vi "CheckTotalSamples.vi"(0 "Digitizer Settings":T1={"Digitizer delay (us) "=0.0, "rf points per line"=0, "lines per plane"=0, "Samp Rate (Hz)"=0.0, "Additional dig delay (us)"=0.0, "Voltage Scale"=0.0, "Pre-Looks"=0, "Offset delay (us)"=0.0, "bits A/D"=0, "Avg Num"=0, "DigTimeOut"=0.0, "Rel Dig Delay"=0.0, "Dig Ch"=0, "LeCroyCluster"={"LeCroy Channels"=[], "LC read pt offset"=0.0, "Sweep Avg"=FALSE}, "Main Digitizer"=enum."Acqiris Digitizer", "Dig Config"=enum."Single channel", "Digitizer ID Cluster"={"Acqiris/Alazar/SP ID"=[], "NI Instr Handles"=[], "LeCroy VISA"="", "GaGe Handle"={"Handle"=0, "Sample size"=0, "Resolution"=0, "Offset"=0, "Channels"=0, "Boards"=0}, "ATS Ref"="ATS9350", "Acqiris Address"=["PCI::INSTR0"], "ADQRef"=refnum, "adq_cu_ptr"=refnum}, "Trigger Settings"={"Trig Source"=1, "Trig Coupling"=0, "Trig Slope"=0, "Level (mV)"=1500.0}, "Bulk Acq"=FALSE, "Bulk Start Indexes"=[], "Data Ref RF"=refnum, "NI ID/Channel"=[], "Total Dig CH"=1, "Xtra Ann Trig delay (us)"=10.0, "Fix Z Delay?"=FALSE, "One Way Transmission?"=FALSE, "Data Ref Log"=refnum} {"Trigger Settings"."Trig Slope" items=["Positive", "Negative"]; "Trigger Settings"."Level (mV)" format="%.2f"; "Trigger Settings"."Trig Coupling" items=["DC 1 MOhm", "AC 1 MOhm", "DC 50 Ohm", "AC 50 Ohm"]; "Trigger Settings"."Trig Source" items=["Chan 1", "External"]; "Rel Dig Delay" format="%.2f"; "DigTimeOut" format="%.2f"; "Avg Num" min=1; "Offset delay (us)" format="%.2f"; "Additional dig delay (us)" format="%.2f"; "Digitizer delay (us)" format="%.2f"}, 1 "Multi Trig":bool, 2 "Multi Trig#":i32, 7 "Valid combo":bool=TRUE, 11 "Bulk Acq":bool) -> (4 "Total Pts":bool=TRUE)   [LabVIEW 2022 SP3]
uses:
  DigitizerSettings.ctl
  Digitizer.ctl
  DigConfig.ctl
  DigitizerID.ctl
  C:/Windows/System32/ADQAPI_dotNet_helper.dll
  <instrlib>/LeCroy Wave Series/LeCroy Wave Series.lvlib
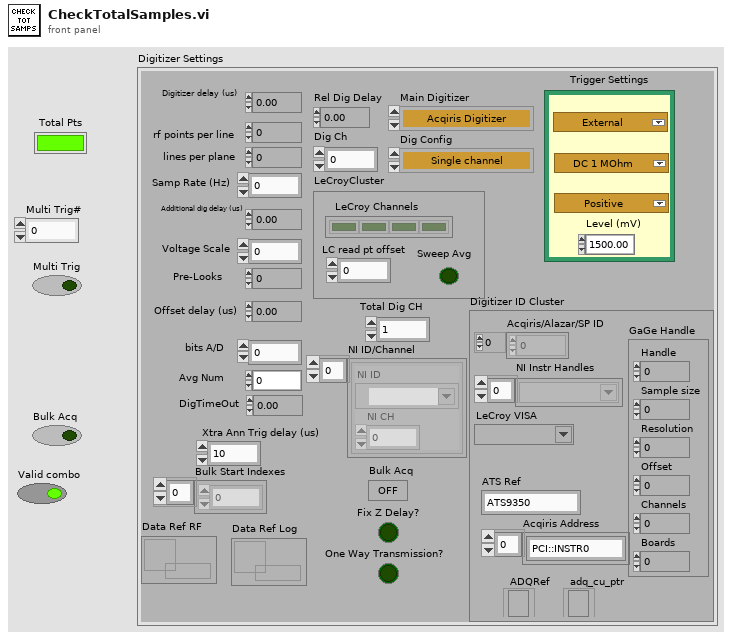
[diagram p1: front panel]
types:
  T1 = typedef "DigitizerSettings.ctl" = cluster{"Digitizer delay (us) ":dbl, "rf points per line":i32, "lines per plane":i32, "Samp Rate (Hz)":dbl, "Additional dig delay (us)":dbl, "Voltage Scale":dbl, "Pre-Looks":i32, "Offset delay (us)":dbl, "bits A/D":i8, "Avg Num":i32, "DigTimeOut":sgl, "Rel Dig Delay":sgl, "Dig Ch":i32, "LeCroyCluster":cluster{"LeCroy Channels":bool[], "LC read pt offset":dbl, "Sweep Avg":bool}, "Main Digitizer":T2, "Dig Config":T3, "Digitizer ID Cluster":T4, "Trigger Settings":cluster{"Trig Source":u16, "Trig Coupling":u16, "Trig Slope":u16, "Level (mV)":dbl}, "Bulk Acq":bool, "Bulk Start Indexes":i32[], "Data Ref RF":refnum<data-value>, "NI ID/Channel":cluster{"NI ID":refnum<k15>, "NI CH":i32}[], "Total Dig CH":i32, "Xtra Ann Trig delay (us)":dbl, "Fix Z Delay?":bool, "One Way Transmission?":bool, "Data Ref Log":refnum<data-value>}
  T2 = typedef "Digitizer.ctl" = enum16{"Acqiris Digitizer", "NI Digitizer", "LeCroy", "GaGe", "AlazarTech", "No Digitizer", "Teledyne"}
  T3 = typedef "DigConfig.ctl" = enum16{"Single channel", "2 Chans w/ 2 Acqiris", "2 Chans w/ 1 Acqiris", "5-CH Pulser New", "5-CH pulser w/ ann array", "5-pass style ann array", "Empty"}
  T4 = typedef "DigitizerID.ctl" = cluster{"Acqiris/Alazar/SP ID":u32[], "NI Instr Handles":refnum<k15>[], "LeCroy VISA":refnum<visa-resource-name>, "GaGe Handle":cluster{"Handle":u32, "Sample size":u32, "Resolution":i32, "Offset":i32, "Channels":u32, "Boards":u32}, "ATS Ref":string, "Acqiris Address":string[], "ADQRef":refnum<k24>, "adq_cu_ptr":refnum<k24>}
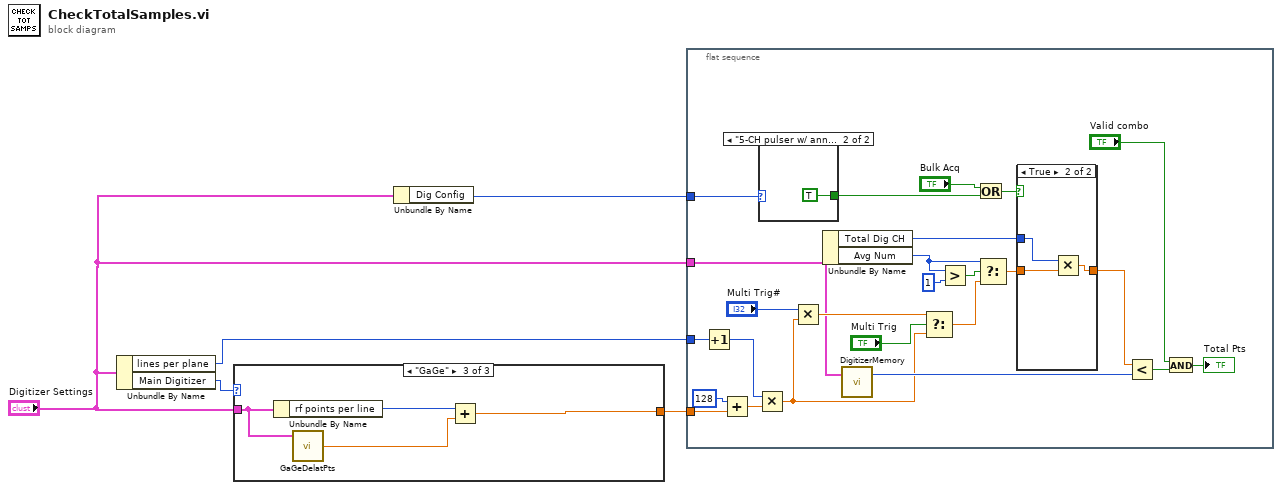
[diagram p0: block diagram]
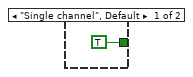
[diagram p2: hidden frame]
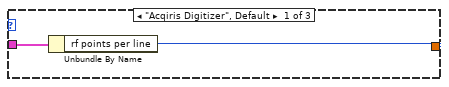
[diagram p4: hidden frame]
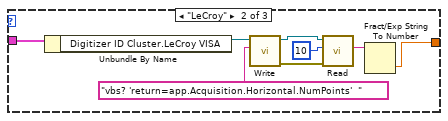
[diagram p5: hidden frame]
diagram:
  n1 = Unbundle By Name("Digitizer Settings") -> ("lines per plane"=w3:i32, "Main Digitizer"=w4:T2)
  n2 = case shown="\"GaGe\"" w4 {
    tunnel: [w6 w11 w18] -> w5
    tunnel: "Digitizer Settings" -> [w7 w8 w16]
    frame "Acqiris Digitizer", Default {
      n3 = Unbundle By Name(w7) -> ("rf points per line"=w6:i32)
    }
    frame "LeCroy" {
      n4 = Unbundle By Name(w8) -> ("Digitizer ID Cluster.LeCroy VISA"=w9:refnum<visa-resource-name>)
      n5 = call <instrlib>:"Write.vi"("Write Buffer"="vbs? 'return=app.Acquisition.Horizontal.NumPoints'  ", "VISA resource name"=w9) -> ("error out"=w14:errorcluster, "VISA resource name out"=w15:refnum<visa-resource-name>)  [unwired: 7 in, 1 out]
      n6 = call <instrlib>:"Read.vi"("error in (no error)"=w14, "Byte Count"=u32 10, "VISA resource name"=w15) -> ("Read Buffer"=w13:string)  [unwired: 5 in, 3 out]
      n7 = Fract/Exp String To Number(string=w13) -> (number=w11:dbl)  [unwired: 3 in, 1 out]
    }
    frame "GaGe" {
      n8 = Unbundle By Name(w16) -> ("rf points per line"=w17:i32)
      n9 = call "GaGeDelatPts.vi"("Digitizer Settings"=w16) -> ("Numeric"=w19:dbl)  [unwired: 4 in]
      n10 = Add(x=w17, y=w19) -> (x+y=w18:dbl)
    }
  }
  n11 = Unbundle By Name("Digitizer Settings") -> ("Dig Config"=w1:T3)
  n12 = flat-sequence {
    tunnel: w5 -> [w41]
    tunnel: w3 -> [w23]
    tunnel: "Digitizer Settings" -> [w22]
    tunnel: w1 -> [w21]
    frame #0 {
      n13 = Increment(x=w23) -> (x+1=w26:i32)
      n14 = Add(x=128, y=w41) -> (x+y=w24:dbl)
      n15 = Multiply(x=w26, y=w24) -> (x*y=w28:dbl)
      n16 = case shown="\"5-CH pulser w/ ann array\", \"5-pass style ann array\"" w21 {
        tunnel: [TRUE TRUE] -> w42
        frame "Single channel", Default {
        }
        frame "5-CH pulser w/ ann array", "5-pass style ann array" {
        }
      }
      n17 = Multiply(x="Multi Trig#", y=w28) -> (x*y=w27:dbl)
      n18 = Unbundle By Name(w22) -> ("Total Dig CH"=w20:i32, "Avg Num"=w43:i32)
      n19 = call "DigitizerMemory.vi"("Digitizer Settings"=w22) -> ("Memory"=w44:i32)  [unwired: 2 out]
      n20 = Select(t=w27, s="Multi Trig", f=w28) -> (s? t:f=w31:dbl)
      n21 = Greater?(x=w43, y=1) -> (0:w30:bool)
      n22 = Or(x="Bulk Acq", y=w42) -> (x .or. y?=w38:bool)
      n23 = Select(t=w43, s=w30, f=w31) -> (s? t:f=w40:dbl)
      n24 = case shown="True" w38 {
        tunnel: w40 -> [w47 w50]
        tunnel: [w47 w49] -> w35
        tunnel: w20 -> [_ w48]
        frame False {
        }
        frame True {
          n25 = Multiply(x=w48, y=w50) -> (x*y=w49:dbl)
        }
      }
      n26 = Less?(x=w35, y=w44) -> (x < y?=w33:bool)
      n27 = And(x="Valid combo", y=w33) -> (x .and. y?=→"Total Pts":bool)
    }
  }
